vi "GEM_BANK_Flatten.vi"(8 "error in (no error)":errorcluster, 11 "LVBANK in":refnum<class "GEM_BANK.lvclass">) -> (0 "error out":errorcluster, 2 "output array":u8[](array[numeric]), 3 "LVBANK out":refnum<class "GEM_BANK.lvclass">)   [LabVIEW 2018, in "feGEM DataPacker.lvlib" / "GEM_BANK.lvclass"]
uses:
  GEM_BANK.lvclass
  GEM_BANK.lvclass/GEM_BANK.ctl
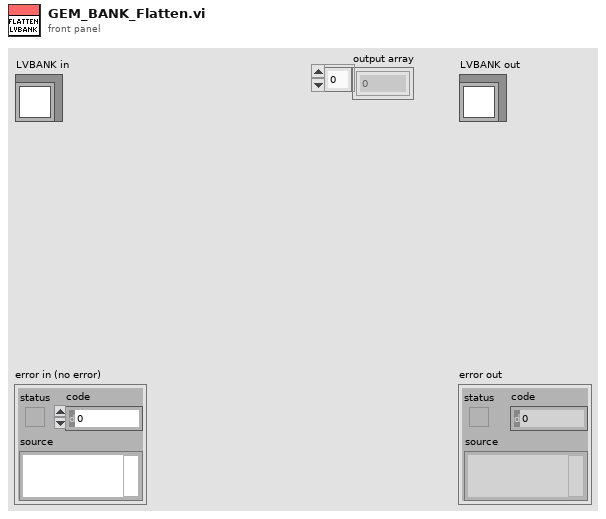
[diagram p1: front panel]
types:
  T1 = enum16{"big-endian, network order", "native, host order", "little-endian"}
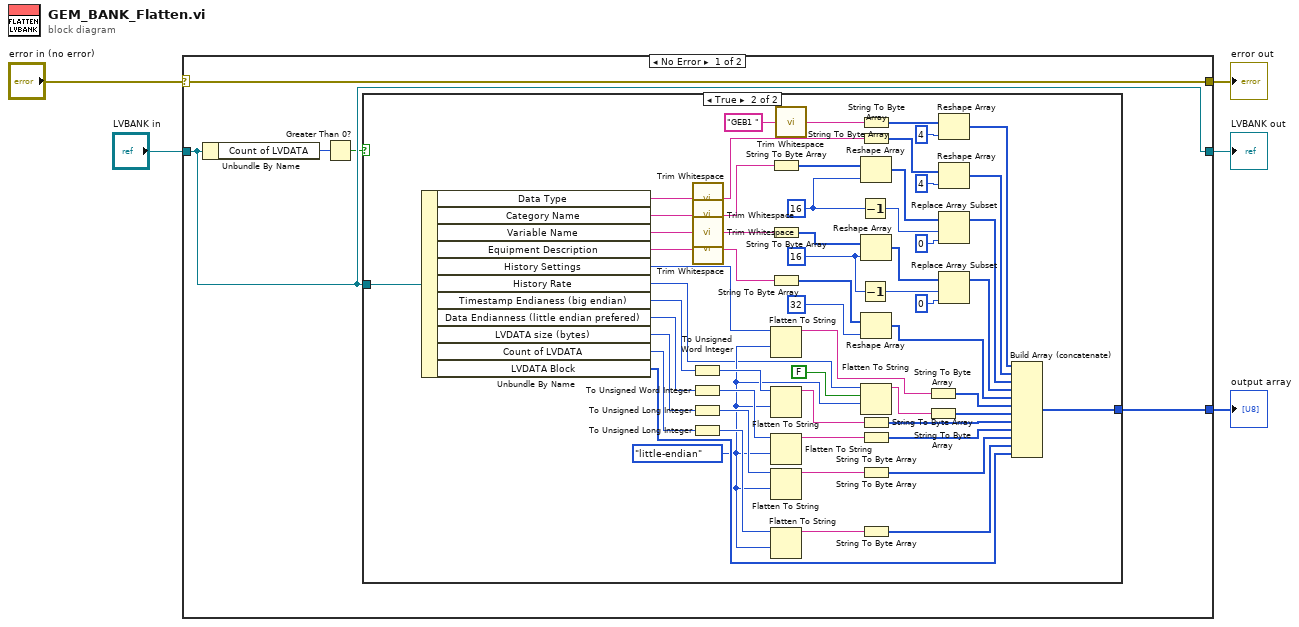
[diagram p0: block diagram]
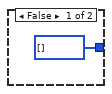
[diagram p2: hidden frame]
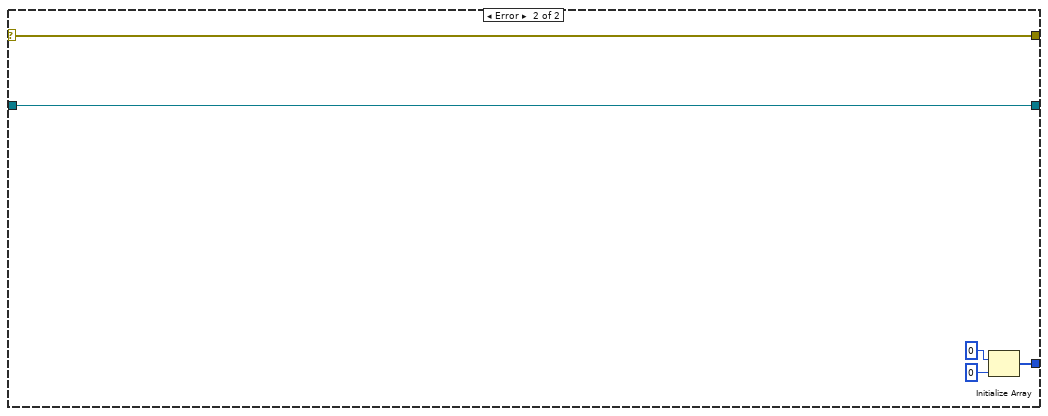
[diagram p3: hidden frame]
diagram:
  n1 = case shown="No Error" "error in (no error)" {
    selector: "error in (no error)" -> [w10 w74]
    tunnel: [w10 w74] -> w4
    tunnel: [w8 w73] -> w3
    tunnel: "LVBANK in" -> [w8 w73]
    tunnel: [w9 w71] -> w2
    frame No Error {
      n2 = Unbundle By Name(w8) -> ("Count of LVDATA"=w7:i32)
      n3 = Greater Than 0?(x=w7) -> (x > 0?=w6:bool)
      n4 = case shown="True" w6 {
        tunnel: w8 -> [_ w69]
        tunnel: [u8[] [] w34] -> w9
        frame False {
        }
        frame True {
          w48 = 16 ("dimension size")
          w52 = 16 ("dimension size")
          w18 = T1."little-endian" ("byte order (0:big-endian, network order)")
          n5 = Unbundle By Name(w69) -> ("Data Type"=w38:string, "Category Name"=w39:string, "Variable Name"=w37:string, "Equipment Description"=w36:string, "History Settings"=w19:u16, "History Rate"=w13:u16, "Timestamp Endianess (big endian)"=w20:T1, "Data Endianness (little endian prefered)"=w21:T1, "LVDATA size (bytes)"=w22:u32, "Count of LVDATA"=w23:i32, "LVDATA Block"=w24:u8[])
          n6 = To Unsigned Word Integer(number=w20) -> (unsigned 16bit integer=w29:u16)
          n7 = To Unsigned Word Integer(number=w21) -> (unsigned 16bit integer=w30:u16)
          n8 = To Unsigned Long Integer(number=w22) -> (unsigned 32bit integer=w67:u32)
          n9 = To Unsigned Long Integer(number=w23) -> (unsigned 32bit integer=w66:u32)
          n10 = call <vilib>:"Trim Whitespace.vi"("string"=w38) -> ("trimmed string"=w55:string)  [unwired: 1 in]
          n11 = call <vilib>:"Trim Whitespace.vi"("string"=w39) -> ("trimmed string"=w64:string)  [unwired: 1 in]
          n12 = call <vilib>:"Trim Whitespace.vi"("string"=w37) -> ("trimmed string"=w61:string)  [unwired: 1 in]
          n13 = call <vilib>:"Trim Whitespace.vi"("string"=w36) -> ("trimmed string"=w45:string)  [unwired: 1 in]
          n14 = String To Byte Array(string=w64) -> (unsigned byte array=w63:u8[])
          n15 = String To Byte Array(string=w61) -> (unsigned byte array=w62:u8[])
          n16 = String To Byte Array(string=w45) -> (unsigned byte array=w46:u8[])
          n17 = Flatten To String(anything=w19, byte order (0:big-endian, network order)=w18) -> (data string=w17:string)  [unwired: 2 in, 2 out]
          n18 = Flatten To String(anything=w29, byte order (0:big-endian, network order)=w18) -> (data string=w28:string)  [unwired: 2 in, 2 out]
          n19 = Flatten To String(anything=w30, byte order (0:big-endian, network order)=w18) -> (data string=w42:string)  [unwired: 2 in, 2 out]
          n20 = Flatten To String(anything=w67, byte order (0:big-endian, network order)=w18) -> (data string=w41:string)  [unwired: 2 in, 2 out]
          n21 = Flatten To String(anything=w66, byte order (0:big-endian, network order)=w18) -> (data string=w40:string)  [unwired: 2 in, 2 out]
          n22 = call <vilib>:"Trim Whitespace.vi"("string"="GEB1 ") -> ("trimmed string"=w58:string)  [unwired: 1 in]
          n23 = Decrement(x=w52) -> (x-1=w51:i32)
          n24 = Decrement(x=w48) -> (x-1=w49:i32)
          n25 = String To Byte Array(string=w58) -> (unsigned byte array=w60:u8[])
          n26 = String To Byte Array(string=w55) -> (unsigned byte array=w57:u8[])
          n27 = Reshape Array(w63, w52) -> (w54:u8[])
          n28 = Reshape Array(w62, w48) -> (w50:u8[])
          n29 = Reshape Array(w46, 32 ("dimension size")) -> (w12:u8[])
          n30 = Flatten To String(anything=w13, prepend array or string size? (T)=FALSE, byte order (0:big-endian, network order)=w18) -> (data string=w43:string)  [unwired: 1 in, 2 out]
          n31 = String To Byte Array(string=w28) -> (unsigned byte array=w16:u8[])
          n32 = String To Byte Array(string=w42) -> (unsigned byte array=w25:u8[])
          n33 = String To Byte Array(string=w41) -> (unsigned byte array=w26:u8[])
          n34 = String To Byte Array(string=w40) -> (unsigned byte array=w27:u8[])
          n35 = String To Byte Array(string=w17) -> (unsigned byte array=w14:u8[])
          n36 = String To Byte Array(string=w43) -> (unsigned byte array=w15:u8[])
          n37 = Reshape Array(w60, 4 ("dimension size")) -> (w31:u8[])
          n38 = Reshape Array(w57, 4 ("dimension size")) -> (w32:u8[])
          n39 = Replace Array Subset(array=w54, new element=u8 0 ("new element/subarray"), index=w51) -> (w33:u8[])
          n40 = Replace Array Subset(array=w50, new element=u8 0 ("new element/subarray"), index=w49) -> (w35:u8[])
          n41 = Build Array (concatenate)(w31, w32, w33, w35, w12, w14, w15, w16, w25, w26, w27, w24) -> (w34:u8[])
        }
      }
    }
    frame Error {
      n42 = Initialize Array(u8 0 ("length (rest)"), 0 ("dimension size")) -> (w71:u8[])
    }
  }
  "error out" <- w4
  "LVBANK out" <- w3
  "output array" <- w2
